vi "Main_07A.vi"() -> ()   [LabVIEW 2025]
uses:
  Utility/Universal Utility/TypeDefs_Utility/Cluster_Row-Column.ctl
  Utility/Universal Utility/TypeDefs_Utility/ENUM_8 Directions U-D-L-R.ctl
  1ebcda4e-5e5e-4b36-b254-ea0519449ada.vi
  e8391653-1ac9-4891-ad08-c1bb4d6ea328.vi
  49602f5a-f202-4fef-abac-66d5f65c7926.vi
  <vilib>/Utility/error.llb/Trim Whitespace.vi
  <vilib>/Utility/error.llb/Trim Whitespace One-Sided.vi
  9e3f57c0-2ef8-4495-8287-c6a42a5fb955.vi
  Utility/Universal Utility/TypeDefs_Utility/ENUM_4 Directions U-D-L-R.ctl
  299cb445-af19-43c4-83da-fdf18fff65e6.vi
panel:
  out "Character Array":string[][](array[string])
  out "MATCH":bool
  in  "Select Data":enum32{"Example", "Puzzle"}(tab)
  in  "EX Target":u64=21
  in  "Example":string=".......S.......\n...............\n.......^.......\n...............\n......^.^......\n...............\n.....^.^.^.....\n...............\n....^.^...^....\n...............\n...^.^...^.^...\n...............\n..^...^.....^..\n...............\n.^.^.^.^.^...^.\n..............."
  in  "Puzzle":string="......................................................................S......................................................................\n.............................................................................................................................................\n......................................................................^......................................................................\n.............................................................................................................................................\n.....................................................................^.^.....................................................................\n.............................................................................................................................................\n....................................................................^...^....................................................................\n.............................................................................................................................................\n...................................................................^.^.^.^...................................................................\n.............................................................................................................................................\n..................................................................^.^.^...^..................................................................\n.............................................................................................................................................\n.................................................................^.^.^.^.^.^.................................................................\n.............................................................................................................................................\n................................................................^.^.^.^.^...^................................................................\n.............................................................................................................................................\n...............................................................^.^.^...^.^.^.^...............................................................\n.............................................................................................................................................\n..............................................................^.^.^.^.^.^...^.^..............................................................\n.............................................................................................................................................\n.............................................................^.^.......^...^.^.^.............................................................\n.............................................................................................................................................\n............................................................^.^.^.^.^...^.^.^.^.^............................................................\n.............................................................................................................................................\n...........................................................^.^.^.^.^.^.^.^...^.^.^...........................................................\n.............................................................................................................................................\n..........................................................^.....^.^.^.^.......^.^.^..........................................................\n.............................................................................................................................................\n.........................................................^...^.^.^.^.^...^.^.^.....^.........................................................\n.............................................................................................................................................\n........................................................^.....^.^.....^.^.^.^.....^.^........................................................\n.............................................................................................................................................\n.......................................................^...^.^.^.......^...^...^.^.^.^.......................................................\n.............................................................................................................................................\n......................................................^.^.^.^.^.^.^.^.^.^.^.^.^...^.^.^......................................................\n.............................................................................................................................................\n.....................................................^.^.^.^...^...^...........^.^.^.^.^.....................................................\n.............................................................................................................................................\n....................................................^.^...^.^.....^.^...^.^.^.^.^...^...^....................................................\n.............................................................................................................................................\n...................................................^.^...^...^...^...^.^.^.^.^...^.^.^.^.^...................................................\n.............................................................................................................................................\n..................................................^.....^.^.....^.^.^.^.^.^...^.^.....^.^.^..................................................\n.............................................................................................................................................\n.................................................^.^.^...^.^.^.....^.^.^.^.^.....^.^.^...^.^.................................................\n.............................................................................................................................................\n................................................^...^...^...^.^.^.........^.^.^.^.^.^.......^................................................\n.............................................................................................................................................\n...............................................^.^.^.^...^.^.^.......^.^.........^.^.^.^.....^...............................................\n.............................................................................................................................................\n..............................................^.^.^...^.^.^.^.^.^...^.^.....^.......^.^.^...^.^..............................................\n.............................................................................................................................................\n.............................................^.^.^.^.^.^...^.^.^.....^.^.^.^.^.^.^.....^.^.^.^.^.............................................\n.............................................................................................................................................\n............................................^.^.^...^.^.^.^.^.^.^...^.^.^.^...^.^.^.^.^.^...^.^.^............................................\n.............................................................................................................................................\n...........................................^.^.^.^.^.^.^.^.^.^...^.^.............^.^.^.........^.^...........................................\n.............................................................................................................................................\n..........................................^.^.^.....^.^.^.^...^.^.^.^.^.^...^.^.^.^.^.^...^.^.^...^..........................................\n.............................................................................................................................................\n.........................................^.^...^.^.^.^.^.^.......^.^...^.^.^.^...^...^.^.^...^.^.^.^.........................................\n.............................................................................................................................................\n........................................^.^.^.^.^.^...^...^.^.^.....^.^.^...^.^.^.^.^.^...^.^.^...^.^........................................\n.............................................................................................................................................\n.......................................^.^.^.^.^.^.^.^.^.^.^.^.^.^...^.^.^.^.......^...^.^...^.^.^...^.......................................\n.............................................................................................................................................\n......................................^.^.^.^...^.^...^.^.^.^.^.^.^.^.^.....^.^...^.^.....^.^.^...^...^......................................\n.............................................................................................................................................\n.....................................^.^.^.^.^.^.^.^...^.^.^...^.....^.^...^.^.^.^.....^.^...^...^.^.^.^.....................................\n.............................................................................................................................................\n....................................^...^.^.^.....^.^.^.^.^...^...^...^.^.^.^.^.^.^...^.^.^.^.^...^...^.^....................................\n.............................................................................................................................................\n...................................^...^...^...^.^.^.....^.^...^.^.^.^.^.....^.^.^.^.^.^.....^...^.^.^...^...................................\n.............................................................................................................................................\n..................................^.^.^.^.^...^.....^.....^.......^.^.....^.^...^...^.^.^...^.....^.^.^.^.^..................................\n.............................................................................................................................................\n.................................^.^.....^.^.^.^.......^.......^.^.^.^.^.^...^.^...^.^.^...^...^.^...^.....^.................................\n.............................................................................................................................................\n................................^.^.^.^.^...^.^.^...^.^.^.^.^.^.^.^...^.^.^.^.....^.^.^.....^.^.^.^...^.....^................................\n.............................................................................................................................................\n...............................^.^...^.^.^...^...^.^.....^.....^.^.^.^...^.....^...^...^...^.^.^.^.^.....^.^.^...............................\n.............................................................................................................................................\n..............................^.^.....^.^.^.^...^.^.^.^.^...^.^.^.^.^.^.^.^.^.^.^.^.......^.^.^.....^...^...^.^..............................\n.............................................................................................................................................\n.............................^.^.^.^.........^.....^.^.^...^...^.^.^.^.^...^...^.^.^.^.^.^.^...^.^.^.^...^.^...^.............................\n.............................................................................................................................................\n............................^.^.^.^.^.^.^.^...^.^.....^.^...^.^.^.^.^.....^.^.^.^...^.^.^.^.^...^...^...^...^.^.^............................\n.............................................................................................................................................\n...........................^.^...^.^.^.^.^.^...^.^.^.....^...^.^.^.^.^...^...^.^...^.^.......^.^.^...^.^.^.^.^.^.^...........................\n.............................................................................................................................................\n..........................^.^...^.^.^.^.^.^.^.........^.^...^.^.^.^.^.^.^.......^.^.^...^.^...^...^.^.^.^.^...^.^.^..........................\n.............................................................................................................................................\n.........................^.....^.^.^.^.^.^...^.^.^.^.....^.^.^...^.^.....^.^.^.^.^.^...^...^.^.....^.^.....^.^.^.^.^.........................\n.............................................................................................................................................\n........................^...^...^.^.^.^.^.^.....^.^.^.^.^.^.^.^.^.^.....^.^...^...^...^.^.^.^.^.^.......^.^.^.^.^...^........................\n.............................................................................................................................................\n.......................^.^.^...^.^.......^.^.^.^.^.^...^.^.......^.^.^...^.^...^.^.^.^.^...^.^.^.^...^.^.^.^.^.^.^.^.^.......................\n.............................................................................................................................................\n......................^.^.^.^...^.^.^.^.^.^.^...^.......^.^...^...^...^...^...^...^.....^...^.^.^.^...^.^.^...^.^.^.^.^......................\n.............................................................................................................................................\n.....................^.^.^...^.^...^.^...^.....^...^.^.^.^.....^.^...^.^.^.^.....^...^.......^.^.^...^.....^.^.^.....^.^.....................\n.............................................................................................................................................\n....................^.^.^.^.^.^.^.^...^.^.^.^.^.^.^.....^...^.^.^.^.^...^.^.^.^.^.^.^...^.^.......^...^.^.^.^.^.^.^.....^....................\n.............................................................................................................................................\n...................^.^.....^.....^...^.^...^...^...^.^.^...^.......^.^...^...^.^.^.^.^.^.^.^...^.^.^.^.^...^.^...^...^.^.^...................\n.............................................................................................................................................\n..................^...^.^.^.^.^.^.^.^.^.^.^.^.....^...^...^...^.^.^.^.^.^.^.^.^...^.....^...^...^.^.^.^.^.....^...^.^.^.^.^..................\n.............................................................................................................................................\n.................^.^.^.^.....^...^.^.^.^.^.^.^.^.^.^...^.^.^.^.^.^.^.....^.^.^...^.^.^...^.......^.....^.^...^...^.......^.^.................\n.............................................................................................................................................\n................^.^...^.....^.^...^.^...^.^.^...^.^.^.^...^.^.^.^.....^.^...^.^...^.^...^.^.....^.^.^.....^.^.^.^.^.^...^...^................\n.............................................................................................................................................\n...............^.^.....^.^.^.^.^.^.^.^...^.^...^.^...^.^.^...^.^.....^.^...^.^.^.^.^.........^.^...^.^.^...^.^.^.....^...^.^.^...............\n.............................................................................................................................................\n..............^.^.^.^.^.^.^.^.^.^.^...^.^.^.^.^.^.^.^.....^.^.^...^.^.^.^.^.^.^.^...^.^.^.^.^.^.^.^.........^.^.^.^.^...^.^.^.^..............\n.............................................................................................................................................\n.............^.^.^.^.^.^...^.^.^.^...^.^.^.^.^.........^.^...^.^.^.....^.^...^.^.^...^.^.^...^.^...^...^...^...^.^.^.^.^.^...^.^.............\n.............................................................................................................................................\n............^.^.....^.^...^.^.^.^.......^.^.^.^.^.....^.^.^.^.^.^.^.^.^.^.^...^.^.^.^.^...^.^.^...^.^...^.^.^...^.^.^.^.^.^.^...^............\n.............................................................................................................................................\n...........^.^.^...^.^.^.^.^...^...^.^.^.....^.^...^.^.^...^.^.^...^.^.^.^...^...^.^.....^...^.^.....^.^.^.^.^.^.^.^...^.......^.^...........\n.............................................................................................................................................\n..........^.^.^.^.^.^...^...^.^.^.^.^.^.....^.^.^.^.^...^...^.^.^...^.^.^.^.^...^.^.^.^.....^.^.^.^.^.^.^.^.^.^.^.....^.^.^.......^..........\n.............................................................................................................................................\n.........^.^.^.^.^...^.^...^...^.....^.^...^.^...^.^.^.^.^.^.........^.^.^.^.^...^.^.^...^.^.^.^.^...^.....^.^.^.^.^.^.^.^.^.^.^...^.........\n.............................................................................................................................................\n........^...^.....^.^.......^...^.^.^.^.....^.^.^.^.......^.^...^.^.^.^.^.^.^.^.^.^.^.....^...^.^.....^...^.^.^.^.^...^...^.....^.^.^........\n.............................................................................................................................................\n.......^.^.^.^.^.^...^.^.^...^.^...^...^.......^.^.^.^.^.^...^.^.^.^.^...^.^.^.^.^.^.^.^.^.^.^...^.^.^.^.^.^.^.^.^.....^.^.^.^...^.^.^.......\n.............................................................................................................................................\n......^.^.^.^.......^.^.^.^.....^.^.^...^.^.^.^.^...^...^...^.^.^.........^.....^.^.^.^.^.^.....^.......^.^.......^.....^.^.^.^.^.....^......\n.............................................................................................................................................\n.....^.^.^.^.....^.^.^...^...^.......^.^...^.....^.^.^.^.^...^...^.^.^.^...^.^.^.^.^.^.^.^.^...^.......^...^.........^.^.^.^...^.^...^.^.....\n.............................................................................................................................................\n....^.^.^.^.^.^.^.^.^.^...^.^...^.^.^...^.^.^.^...^.^...^.^.^.^...^...^.^.^.^.^.^.^...^.^.^...^.......^.^.^.^.^.^.^.^.^.^.^.^...^.^.^...^....\n.............................................................................................................................................\n...^...^.^.^.^...^.^...^.^.....^.^.^.^.^.^.^.^.^.....^.^.^...^...^.^.^.^.^...^...^.^.^.^...^.^.^.^.^...^...^.^.^.^.^...^.^.^.^.....^.....^...\n.............................................................................................................................................\n..^.^...^...^.^.^.^...^.^.^...^.^.^.^.^.....^...^...^.^.^.....^.^.....^.^.^...^.....^.^...^.^.^.^...^.......^.^.....^.^.......^.^.......^.^..\n.............................................................................................................................................\n.^...^.^.^.^.^.^.....^.^.^.........^.^...^.^.^.^...^.^.^.^...^.^.........^.^...^.....^...^.^.^.^.^.^.^...^...^.^.^.........^.^.^.^.^.^.^.^.^.\n............................................................................................................................................."
  in  "Puzzle Target":u64=1635
  out "Answer":u64
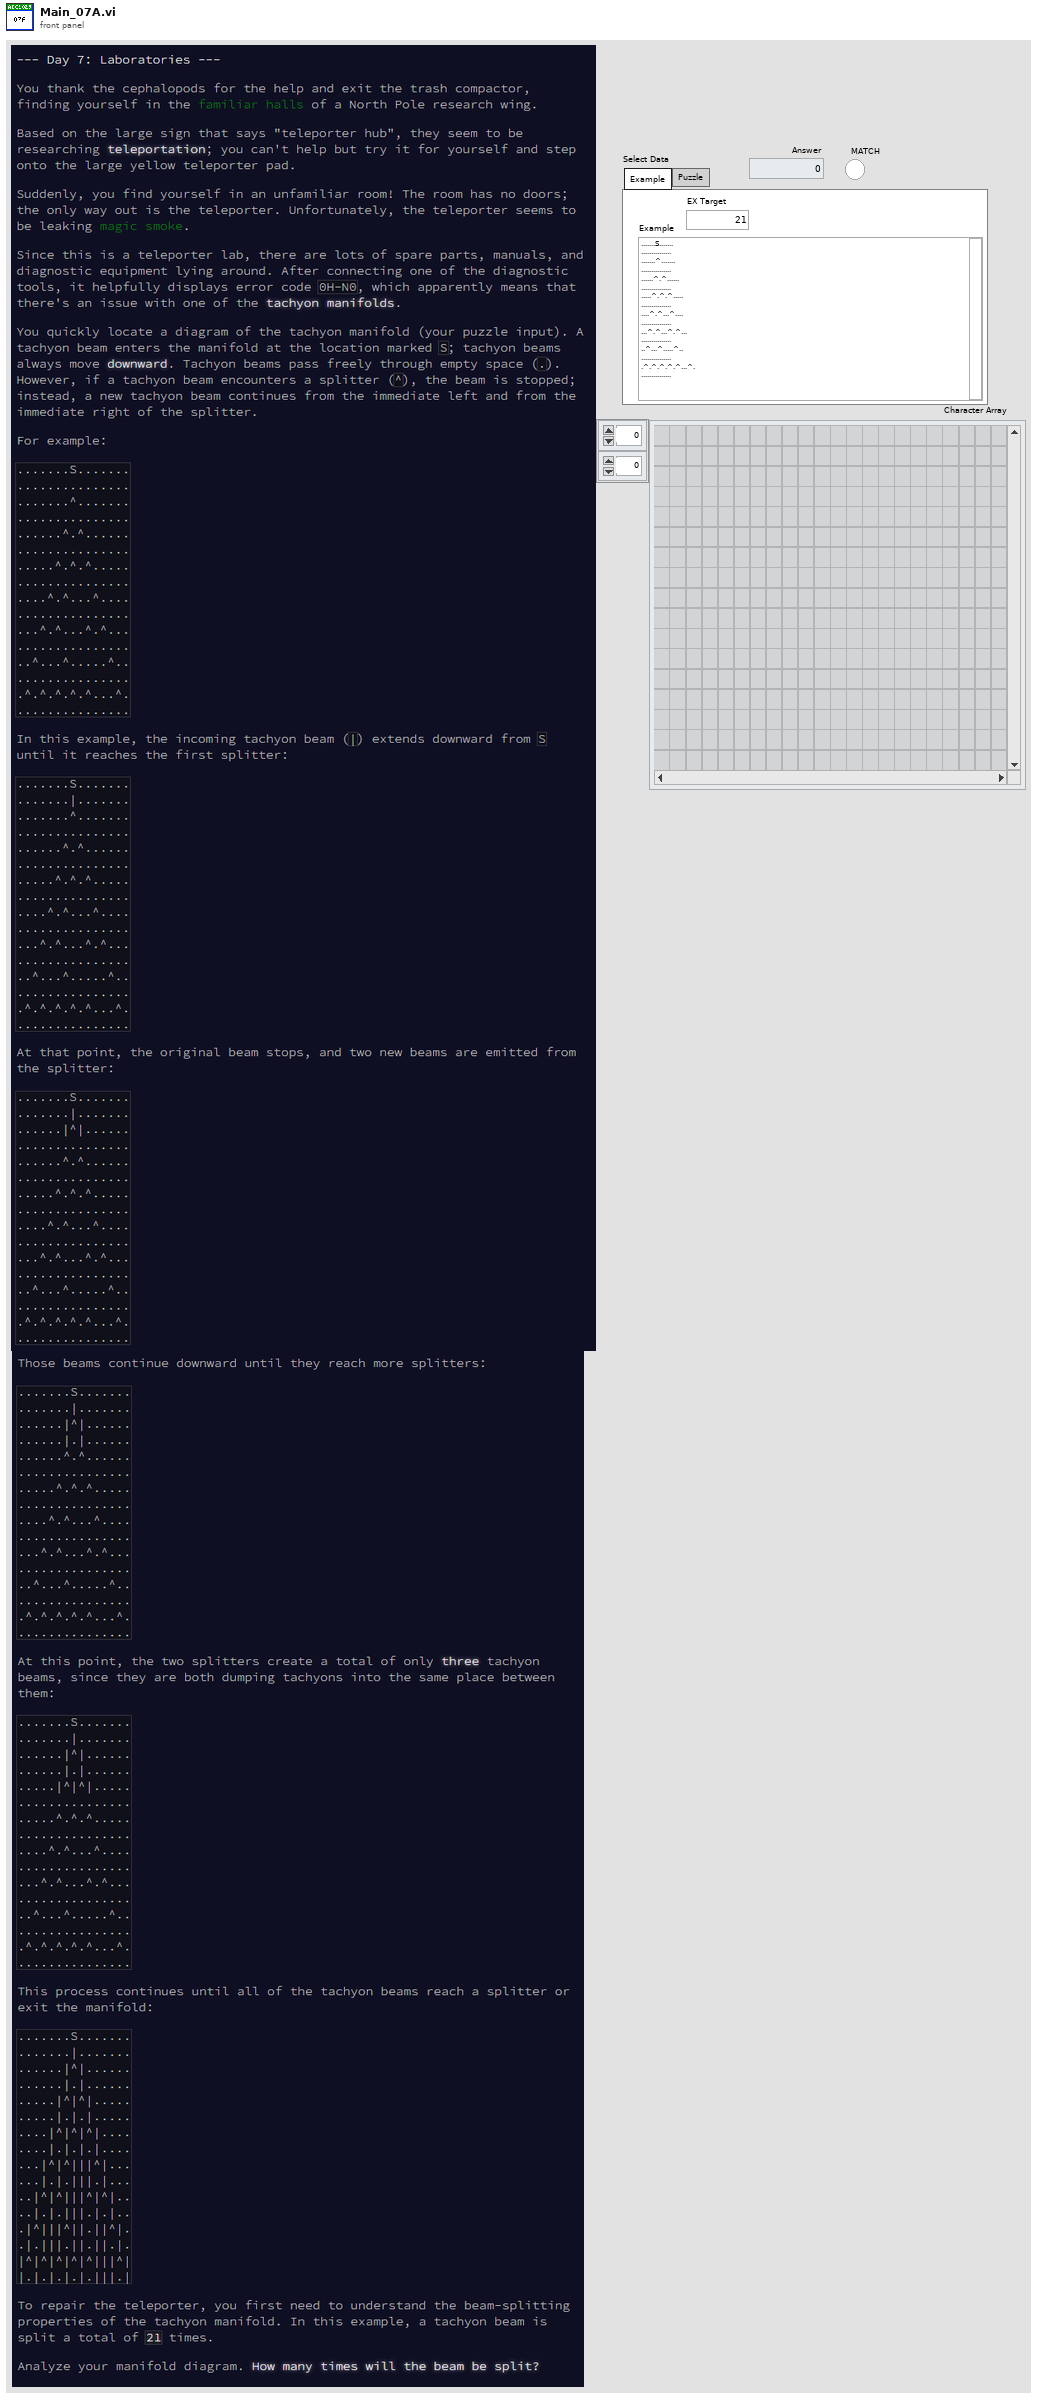
[diagram p1: front panel]
types:
  T1 = typedef "Cluster_Row-Column.ctl" = cluster{"R":i32, "C":i32}
  T2 = typedef "ENUM_8 Directions U-D-L-R.ctl" = enum16{"Up;-1,0", "Up-Right;-1,1", "Right;0,1", "Down-Right;1,1", "Down;1,0", "Down-Left;1,-1", "Left;0,-1", "Up-Left;-1,-1"}
  T3 = typedef "ENUM_4 Directions U-D-L-R.ctl" = enum16{"Up;-1,0", "Right;0,1", "Down;1,0", "Left;0,-1"}
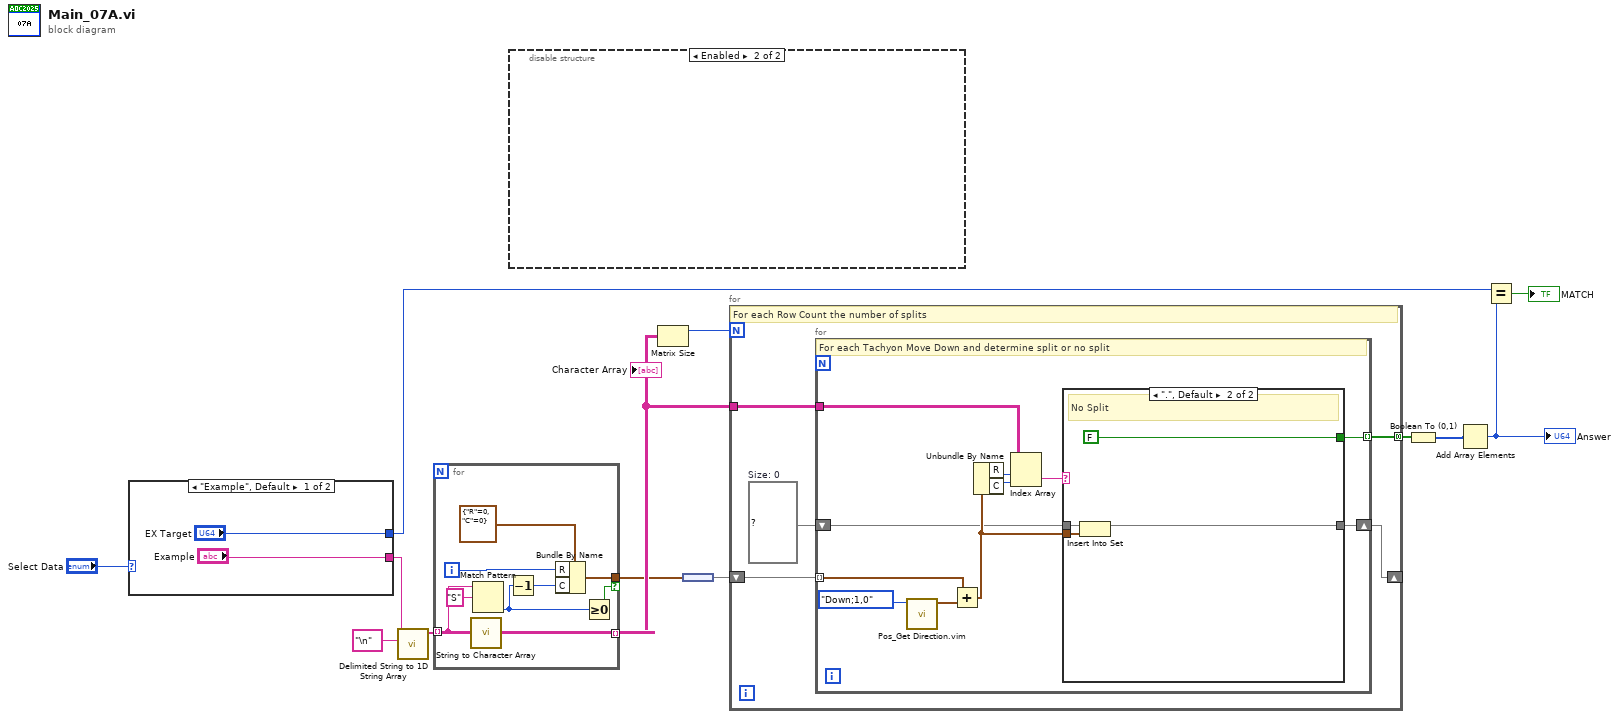
[diagram p0: block diagram]
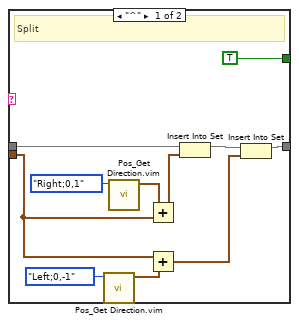
[diagram p2: hidden frame]
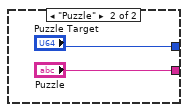
[diagram p3: hidden frame]
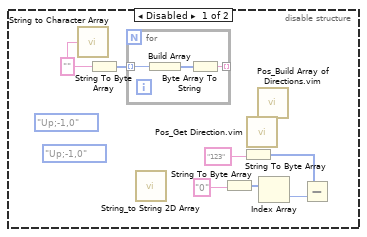
[diagram p4: hidden frame]
diagram:
  n1 = case shown="\"Example\", Default" "Select Data" {
    tunnel: ["Example" "Puzzle"] -> w11
    tunnel: ["EX Target" "Puzzle Target"] -> w8
    frame "Example", Default {
    }
    frame "Puzzle" {
    }
  }
  n2 = call <vilib>:"Delimited String to 1D String Array.vi"("delimiter"="\n" ("delimiter (Tab)"), "delimited string"=w11) -> ("string array"=w12:string[])  [unwired: 9 in]
  n3 = for {
    tunnel: w12 -> [w25] mode=indexing
    tunnel: [w26] -> w7 mode=indexing
    tunnel: [w20] -> w5 if=w19
    i -> [w22]
    n4 = call "String to Character Array.vi"("Input String"=w25) -> ("Character Array"=w26:string[])
    n5 = Match Pattern(string=w25, regular expression="S") -> (offset past match=w21:i32)  [unwired: 1 in, 3 out]
    n6 = Decrement(x=w21) -> (x-1=w18:i32)
    n7 = Bundle By Name(cluster=T1 {"R"=0, "C"=0} ("Position"), "R"=w22, "C"=w18) -> (w20:T1)
    n8 = Greater Or Equal To 0?(x=w21) -> (x >= 0?=w19:bool)
  }
  "Character Array" <- w7
  n9 = disable-structure shown="Enabled" {
    frame Disabled {
      w29 = "" ("string")
      (unwired) ENUM_8_Directions_U-D-L-R."Up;-1,0" ("Direction 8")
      (unwired) ENUM_4_Directions_U-D-L-R."Up;-1,0" ("Direction")
      n10 = call "String to Character Array.vi"("Input String"=w29) -> ()  [unwired: 1 out]
      n11 = String To Byte Array(string=w29) -> (unsigned byte array=w30:u8[])
      n12 = for {
        tunnel: w30 -> [w36] mode=indexing
        tunnel: [w34] -> _ mode=indexing
        n13 = Build Array(w36) -> (w35:u8[])
        n14 = Byte Array To String(unsigned byte array=w35) -> (string=w34:string)
      }
      n15 = call "String_to String 2D Array.vi"() -> ()  [unwired: 11 in, 1 out]
      n16 = String To Byte Array(string="0") -> (unsigned byte array=w33:u8[])
      n17 = String To Byte Array(string="123") -> (unsigned byte array=w31:u8[])
      n18 = call "Pos_Get Direction.vim"() -> ()  [unwired: 11 in, 1 out]
      n19 = call "Pos_Build Array of Directions.vim"() -> ()  [unwired: 10 in, 2 out]
      n20 = Index Array(array=w33) -> (element=w32:u8)  [unwired: 1 in]
      n21 = Subtract(x=w31, y=w32) -> ()  [unwired: 1 out]
    }
    frame Enabled {
    }
  }
  n22 = Matrix Size(0:w7) -> (1:w6:i32)  [unwired: 1 out]
  n23 = node(w5) -> (w4:set{T1})
  n24 = for {
    N: w6 -> [_]
    tunnel: w7 -> [w40]
    shift-right: [w38] -> _
    shift-left: w4 -> [w41]
    tunnel: [w37] -> w3 mode=concatenating
    w39 = set{T1} {}  # Size: 0
    # "For each Row Count the number of splits"
    n25 = for {
      tunnel: w41 -> [w50] mode=indexing
      tunnel: w40 -> [w49]
      shift-right: [w43] -> w38
      shift-left: w39 -> [w44]
      tunnel: [w42] -> w37 mode=indexing
      # "For each Tachyon Move Down and determine split or no split"
      n26 = call "Pos_Get Direction.vim"("Direction 8"=ENUM_8_Directions_U-D-L-R."Down;1,0") -> ("Position"=w51:T1)  [unwired: 10 in]
      n27 = Add(x=w50, y=w51) -> (x+y=w45:T1)
      n28 = Unbundle By Name(w45) -> ("R"=w48:i32, "C"=w47:i32)
      n29 = Index Array(array=w49, index (row)=w48, index (col)=w47) -> (element=w46:string)
      n30 = case shown="\".\", Default" w46 {
        tunnel: w45 -> [w60 w66]
        tunnel: w44 -> [w58 w67]
        tunnel: [w55 w65] -> w43
        tunnel: [TRUE FALSE] -> w42
        frame "^" {
          # "Split"
          n31 = call "Pos_Get Direction.vim"("Direction 8"=ENUM_8_Directions_U-D-L-R."Left;0,-1") -> ("Position"=w59:T1)  [unwired: 10 in]
          n32 = call "Pos_Get Direction.vim"("Direction 8"=ENUM_8_Directions_U-D-L-R."Right;0,1") -> ("Position"=w61:T1)  [unwired: 10 in]
          n33 = Add(x=w61, y=w60) -> (x+y=w57:T1)
          n34 = Add(x=w60, y=w59) -> (x+y=w54:T1)
          n35 = Insert Into Set(10:w57, 11:w58) -> (3:w56:set{T1})  [unwired: 1 out]
          n36 = Insert Into Set(10:w54, 11:w56) -> (3:w55:set{T1})  [unwired: 1 out]
        }
        frame ".", Default {
          # "No Split"
          n37 = Insert Into Set(10:w66, 11:w67) -> (3:w65:set{T1})  [unwired: 1 out]
        }
      }
    }
  }
  n38 = Boolean To (0,1)(Boolean=w3) -> (0, 1=w2:i16[])
  n39 = Add Array Elements(numeric array=w2) -> (sum=w1:i16)
  "Answer" <- w1
  n40 = Equal?(x=w8, y=w1) -> (x = y?=→"MATCH":bool)
